vi "Communication Manager.vi"(7 "Mode":T1(ring)=enum."Get References", 8 "error in":errorcluster, 9 "Error Queue":refnum<queue>, 11 "Application Events":refnum<user-event>) -> (0 "error out":errorcluster, 1 "Error Queue Out":refnum<queue>, 2 "Module Queue Out":refnum<queue>, 3 "Application Events Out":refnum<user-event>)   [LabVIEW 2020, in "User Console.lvlib"]
doc: "Holds reference to communication structure need by the current module both for internal and external use"
uses:
  User Console.lvlib
  Error/Controls/Error Message Object.ctl
  Controller/Controls/Application Modules.ctl
  Error/Controls/Error Commands.ctl
  Controller/Controls/Application Event Object.ctl
  Controller/Controls/Application Events.ctl
  Controls/Operational Loop Message Object.ctl
  Controls/Operational Loop Commands.ctl
  Controller/Controller.lvlib
  Error/Error Handler.lvlib
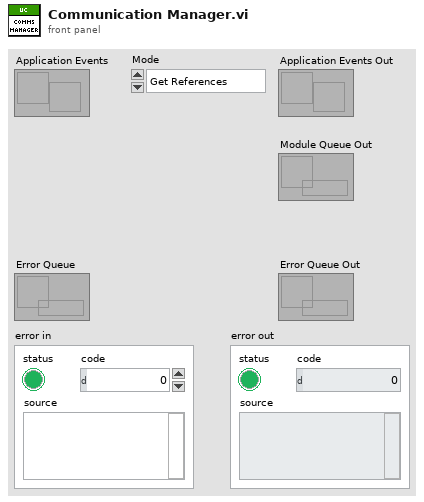
[diagram p1: front panel]
types:
  T1 = enum16{"Load References", "Release References", "Get References"}
  T2 = typedef "User Console.lvlib/Operational Loop Message Object.ctl" = cluster{"Commands":T3, "Source Module":T4, "Event Data":variant}
  T3 = typedef "User Console.lvlib/Operational Loop Commands.ctl" = enum16{"Shutdown"}
  T4 = typedef "Controller.lvlib/Application Modules.ctl" = enum16{"Controller", "Error Module", "User Console", "Display Console", "Sensor Interface"}
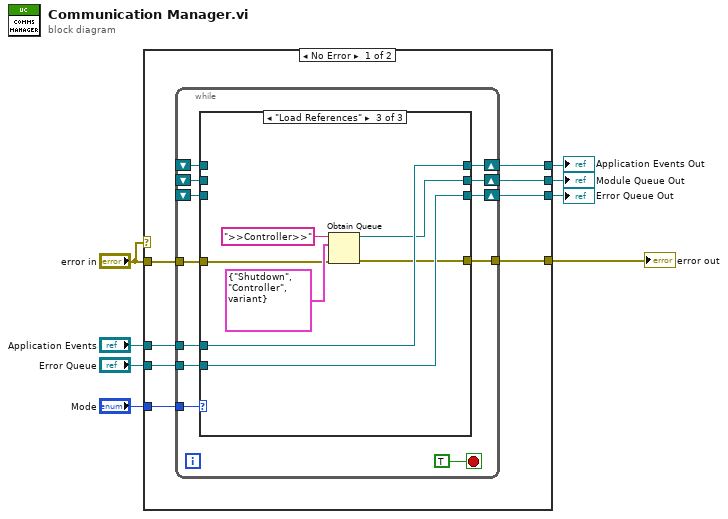
[diagram p0: block diagram]
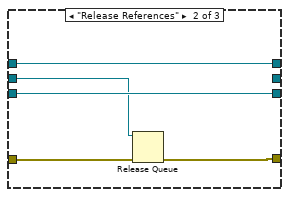
[diagram p3: hidden frame]
diagram:
  n1 = case shown="No Error" "error in" {
    tunnel: [w13 w45] -> w8
    tunnel: "error in" -> [w14 w45]
    tunnel: "Application Events" -> [w16 _]
    tunnel: "Error Queue" -> [w15 _]
    tunnel: [w12 _] -> w4
    tunnel: [w11 _] -> w3
    tunnel: [w10 _] -> w2
    tunnel: "Mode" -> [w9 _]
    frame No Error {
      n2 = while {
        tunnel: w16 -> [w26]
        shift-right: [w27] -> w11
        shift-left: _ -> [w25]
        shift-right: [w23] -> w12
        shift-left: _ -> [w24]
        shift-right: [w22] -> w10
        shift-left: _ -> [w21]
        tunnel: w15 -> [w20]
        tunnel: w14 -> [w19]
        tunnel: [w18] -> w13
        tunnel: w9 -> [w17]
        stop <- TRUE stop-if-true
        n3 = case shown="\"Load References\"" w17 {
          tunnel: [w31 w37 w42] -> w27
          tunnel: w26 -> [_ _ w42]
          tunnel: w25 -> [w31 w37 _]
          tunnel: [w30 _ w41] -> w23
          tunnel: w24 -> [w30 w33 _]
          tunnel: [w29 w36 w40] -> w22
          tunnel: w21 -> [w29 w36 _]
          tunnel: w20 -> [_ _ w40]
          tunnel: w19 -> [w32 w35 w39]
          tunnel: [w32 w34 w38] -> w18
          frame Default {
          }
          frame "Release References" {
            n4 = Release Queue(queue=w33, error in (no error)=w35) -> (error out=w34:errorcluster)  [unwired: 1 in, 2 out]
          }
          frame "Load References" {
            n5 = Obtain Queue(name (unnamed)=">>Controller>>", element data type=T2 {"Commands"=enum."Shutdown", "Source Module"=enum."Controller", "Event Data"=variant} ("Controller Message Object"), error in (no error)=w39) -> (queue out=w41:refnum<queue>, error out=w38:errorcluster)  [unwired: 2 in, 1 out]
          }
        }
      }
    }
    frame Error {
    }
  }
  "error out" <- w8
  "Application Events Out" <- w3
  "Error Queue Out" <- w2
  "Module Queue Out" <- w4
